vi "rsscope_core_global.vi"() -> ()   [LabVIEW 2018] (continued)
"Descriptive Name"="Amplitude Time Arithmetic Parameter Amptime Type", "Data Type"=0, "Command"="MEAS{Measurement}:AMPT:ARIT:PAR{ArithmeticParameter}:AMPT", "Access"=2, "Range Table"="RsScope_rngAmplitudeTimeArithmeticParameterMeasurementType", "Read Callback"="", "Write Callback"="", "Supported Models"="", "Instrument Options"="", "Flags"=0, "Help"="Selects the amplitude/time arithmetics measurements for the measurment group.\n\nAvailable Repeated Capabilities:\nMeasurement: Meas1, Meas2, Meas3, Meas4, Meas5, Meas6, Meas7, Meas8, Meas9, Meas10\r\nArithmeticParameter: ArithmeticParm1, ArithmeticParm2\r\n\nRemote-control command(s):\nMEASurement<m>:AMPTime:ARIThmetic:PARameter<n>:AMPTime"}, {"Level"=4, "Class Only"=FALSE, "Identifier"="RSSCOPE_ATTR_AMPLITUDE_TIME_ARITHMETIC_PARAMETER_GROUP", "Descriptive Name"="Amplitude Time Arithmetic Parameter Group", "Data Type"=0, "Command"="MEAS{Measurement}:AMPT:ARIT:PAR{ArithmeticParameter}:GRO", "Access"=2, "Range Table"="RsScope_rngSpectrumArithmeticParameterGroup", "Read Callback"="", "Write Callback"="", "Supported Models"="", "Instrument Options"="", "Flags"=0, "Help"="Sets the measurement group for the second operand of the amplitude/time arithmetic measurement.\n\nAvailable Repeated Capabilities:\nMeasurement: Meas1, Meas2, Meas3, Meas4, Meas5, Meas6, Meas7, Meas8, Meas9, Meas10\r\nArithmeticParameter: ArithmeticParm1, ArithmeticParm2\r\n\nRemote-control command(s):\nMEASurement<m>:AMPTime:ARIThmetic:PARameter<n>:GROup"}, {"Level"=4, "Class Only"=FALSE, "Identifier"="RSSCOPE_ATTR_AMPLITUDE_TIME_ARITHMETIC_PARAMETER_MEASUREMENT_SPECTRUM", "Descriptive Name"="Amplitude Time Arithmetic Parameter Measurement Spectrum", "Data Type"=0, "Command"="MEAS{Measurement}:AMPT:ARIT:PAR{ArithmeticParameter}:SPEC", "Access"=2, "Range Table"="RsScope_rngSpectrumArithmeticMeasurementSpectrum", "Read Callback"="", "Write Callback"="", "Supported Models"="", "Instrument Options"="", "Flags"=0, "Help"="Selects the spectrum arithmetics measurements for the measurment group.\n\nAvailable Repeated Capabilities:\nMeasurement: Meas1, Meas2, Meas3, Meas4, Meas5, Meas6, Meas7, Meas8, Meas9, Meas10\r\nArithmeticParameter: ArithmeticParm1, ArithmeticParm2\r\n\nRemote-control command(s):\nMEASurement<m>:AMPTime:ARIThmetic:PARameter<n>:SPECtrum"}, {"Level"=4, "Class Only"=FALSE, "Identifier"="RSSCOPE_ATTR_AMPLITUDE_TIME_ARITHMETIC_OPERATOR", "Descriptive Name"="Amplitude Time Arithmetic Operator", "Data Type"=0, "Command"="MEAS{Measurement}:AMPT:ARIT:OPER", "Access"=2, "Range Table"="RsScope_rngSpectrumArithmeticOperator", "Read Callback"="", "Write Callback"="", "Supported Models"="", "Instrument Options"="", "Flags"=0, "Help"="Selects the operation type to be performed on the selected operands for the amplitude/time arithmetic measurement.\n\nAvailable Repeated Capabilities:\nMeasurement: Meas1, Meas2, Meas3, Meas4, Meas5, Meas6, Meas7, Meas8, Meas9, Meas10\r\n\nRemote-control command(s):\nMEASurement<m>:AMPTime:ARIThmetic:OPERator"}, {"Level"=4, "Class Only"=FALSE, "Identifier"="RSSCOPE_ATTR_AMPLITUDE_TIME_ARITHMETIC_CONSTANT", "Descriptive Name"="Amplitude Time Arithmetic Constant", "Data Type"=1, "Command"="MEAS{Measurement}:AMPT:ARIT:CONS", "Access"=2, "Range Table"="RsScope_rngArithmeticConstant", "Read Callback"="", "Write Callback"="", "Supported Models"="", "Instrument Options"="", "Flags"=0, "Help"="Sets a constant numeric value as the second operand of the amplitude/time arithmetic measurement.\n\nAvailable Repeated Capabilities:\nMeasurement: Meas1, Meas2, Meas3, Meas4, Meas5, Meas6, Meas7, Meas8, Meas9, Meas10\r\n\nRemote-control command(s):\nMEASurement<m>:AMPTime:ARIThmetic:CONStant"}, {"Level"=4, "Class Only"=FALSE, "Identifier"="RSSCOPE_ATTR_AMPLITUDE_TIME_ARITHMETIC_CONSTANT_UNIT", "Descriptive Name"="Amplitude Time Arithmetic Constant Unit", "Data Type"=0, "Command"="MEAS{Measurement}:AMPT:ARIT:COUN", "Access"=2, "Range Table"="RsScope_rngArithmeticOperationType", "Read Callback"="", "Write Callback"="", "Supported Models"="", "Instrument Options"="", "Flags"=0, "Help"="Selects the operation type to be performed on the selected operands for the amplitude/time arithmetic measurement.\n\nAvailable Repeated Capabilities:\nMeasurement: Meas1, Meas2, Meas3, Meas4, Meas5, Meas6, Meas7, Meas8, Meas9, Meas10\r\n\nRemote-control command(s):\nMEASurement<m>:AMPTime:ARIThmetic:COUNit"}, {"Level"=4, "Class Only"=FALSE, "Identifier"="RSSCOPE_ATTR_AMPLITUDE_TIME_ARITHMETIC_CUSTOM_NAME_ENABLED", "Descriptive Name"="Amplitude Time Arithmetic Custom Name Enabled", "Data Type"=3, "Command"="MEAS{Measurement}:AMPT:ARIT:CUNS", "Access"=2, "Range Table"="", "Read Callback"="", "Write Callback"="", "Supported Models"="", "Instrument Options"="", "Flags"=0, "Help"="Enables the use of user-defined custom name for the amplitude/time arithmetic measurement.\n\nAvailable Repeated Capabilities:\nMeasurement: Meas1, Meas2, Meas3, Meas4, Meas5, Meas6, Meas7, Meas8, Meas9, Meas10\r\n\nRemote-control command(s):\nMEASurement<m>:AMPTime:ARIThmetic:CUNState"}, {"Level"=4, "Class Only"=FALSE, "Identifier"="RSSCOPE_ATTR_AMPLITUDE_TIME_ARITHMETIC_CUSTOM_UNIT_ENABLED", "Descriptive Name"="Amplitude Time Arithmetic Custom Unit Enabled", "Data Type"=3, "Command"="MEAS{Measurement}:AMPT:ARIT:CUUS", "Access"=2, "Range Table"="", "Read Callback"="", "Write Callback"="", "Supported Models"="", "Instrument Options"="", "Flags"=0, "Help"="Enables the use of user-defined custom unit for the amplitude/time arithmetic measurement. You can set the unit with RSSCOPE_ATTR_AMPLITUDE_TIME_ARITHMETIC_CUSTOM_UNIT.\n\nAvailable Repeated Capabilities:\nMeasurement: Meas1, Meas2, Meas3, Meas4, Meas5, Meas6, Meas7, Meas8, Meas9, Meas10\r\n\nRemote-control command(s):\nMEASurement<m>:AMPTime:ARIThmetic:CUUState"}, {"Level"=4, "Class Only"=FALSE, "Identifier"="RSSCOPE_ATTR_AMPLITUDE_TIME_ARITHMETIC_CUSTOM_UNIT", "Descriptive Name"="Amplitude Time Arithmetic Custom Unit", "Data Type"=2, "Command"="MEAS{Measurement}:AMPT:ARIT:CUUN", "Access"=2, "Range Table"="", "Read Callback"="", "Write Callback"="", "Supported Models"="", "Instrument Options"="", "Flags"=0, "Help"="Sets a user-defined value of the unit for the amplitude/time arithmetic measurement.\n\nAvailable Repeated Capabilities:\nMeasurement: Meas1, Meas2, Meas3, Meas4, Meas5, Meas6, Meas7, Meas8, Meas9, Meas10\r\n\nRemote-control command(s):\nMEASurement<m>:AMPTime:ARIThmetic:CUUNit"}, {"Level"=3, "Class Only"=TRUE, "Identifier"="", "Descriptive Name"="Source Number", "Data Type"=0, "Command"="", "Access"=0, "Range Table"="", "Read Callback"="", "Write Callback"="", "Supported Models"="", "Instrument Options"="", "Flags"=0, "Help"="Selects Source Number"}, {"Level"=4, "Class Only"=FALSE, "Identifier"="RSSCOPE_ATTR_AMPT_DELAY_LEVEL_SELECTION", "Descriptive Name"="Amplitude Delay Level Selection", "Data Type"=0, "Command"="MEAS{Measurement}:AMPT:DEL{SourceNumber}:LSEL", "Access"=2, "Range Table"="rsscope_rngAmpRefLevSelection", "Read Callback"="", "Write Callback"="", "Supported Models"="", "Instrument Options"="", "Flags"=0, "Help"="Selects the reference level on which the time is measured for each source.\n\nAvailable Repeated Capabilities:\nMeasurement: Meas1, Meas2, Meas3, Meas4, Meas5, Meas6, Meas7, Meas8, Meas9, Meas10\r\nSourceNumber: SN1, SN2, SN3, SN4\r\n\nRemote-control command(s):\nMEASurement<m>:AMPTime:DELay<n>:LSELect"}, {"Level"=4, "Class Only"=FALSE, "Identifier"="RSSCOPE_ATTR_AMPT_DELAY_SLOPE", "Descriptive Name"="Amplitude Delay Slope", "Data Type"=0, "Command"="MEAS{Measurement}:AMPT:DEL{SourceNumber}:SLOP", "Access"=2, "Range Table"="rsscope_rngTriggerSlope", "Read Callback"="", "Write Callback"="", "Supported Models"="", "Instrument Options"="", "Flags"=0, "Help"="Sets the edge of each source, between which the delay is measured.\n\nAvailable Repeated Capabilities:\nMeasurement: Meas1, Meas2, Meas3, Meas4, Meas5, Meas6, Meas7, Meas8, Meas9, Meas10\r\nSourceNumber: SN1, SN2, SN3, SN4\r\n\nRemote-control command(s):\nMEASurement<m>:AMPTime:DELay<n>:SLOPe"}, {"Level"=4, "Class Only"=FALSE, "Identifier"="RSSCOPE_ATTR_AMPT_DELAY_DIRECTION", "Descriptive Name"="Amplitude Delay Direction", "Data Type"=0, "Command"="MEAS{Measurement}:AMPT:DEL{SourceNumber}:DIR", "Access"=2, "Range Table"="rsscope_rngAmplitudeDelayDirection", "Read Callback"="", "Write Callback"="", "Supported Models"="", "Instrument Options"="", "Flags"=0, "Help"="Selects the direction for counting slopes for each source: from the beginning of the waveform, or from the end.\n\nAvailable Repeated Capabilities:\nMeasurement: Meas1, Meas2, Meas3, Meas4, Meas5, Meas6, Meas7, Meas8, Meas9, Meas10\r\nSourceNumber: SN1, SN2, SN3, SN4\r\n\nRemote-control command(s):\nMEASurement<m>:AMPTime:DELay<n>:DIRection"}, {"Level"=4, "Class Only"=FALSE, "Identifier"="RSSCOPE_ATTR_AMPT_DELAY_EDGE_NUMBER", "Descriptive Name"="Amplitude Delay Edge Number", "Data Type"=0, "Command"="MEAS{Measurement}:AMPT:DEL{SourceNumber}:ECO", "Access"=2, "Range Table"="rsscope_rngAmpDelayEdgeNumber", "Read Callback"="", "Write Callback"="", "Supported Models"="", "Instrument Options"="", "Flags"=0, "Help"="Sets the number of the edge that is relevant for delay measurement for each source.\n\nAvailable Repeated Capabilities:\nMeasurement: Meas1, Meas2, Meas3, Meas4, Meas5, Meas6, Meas7, Meas8, Meas9, Meas10\r\nSourceNumber: SN1, SN2, SN3, SN4\r\n\nRemote-control command(s):\nMEASurement<m>:AMPTime:DELay<n>:ECOunt"}, {"Level"=3, "Class Only"=TRUE, "Identifier"="", "Descriptive Name"="Amplitude Measurement Type", "Data Type"=0, "Command"="", "Access"=0, "Range Table"="", "Read Callback"="", "Write Callback"="", "Supported Models"="", "Instrument Options"="", "Flags"=0, "Help"="Selects Amplitude Measurement Type"}, {"Level"=4, "Class Only"=FALSE, "Identifier"="RSSCOPE_ATTR_AMPT_LIMIT_CHECK", "Descriptive Name"="Amplitude Time Limit Check", "Data Type"=0, "Command"="MEAS{Measurement}:AMPT:LCH{AmptMeasurementType}:VAL", "Access"=2, "Range Table"="rsscope_rngLimitCheck", "Read Callback"="", "Write Callback"="", "Supported Models"="", "Instrument Options"="", "Flags"=0, "Help"="Enables or disables limit checking for amplitude vs. time measurements in the specified measurement channel.\n\nAvailable Repeated Capabilities:\nMeasurement: Meas1, Meas2, Meas3, Meas4, Meas5, Meas6, Meas7, Meas8, Meas9, Meas10\r\nAmptMeasurementType: Ampt1, Ampt2, Ampt3, Ampt4, Ampt5, Ampt6, Ampt7, Ampt8, Ampt9, Ampt10, Ampt11, Ampt12, Ampt13, Ampt14, Ampt15, Ampt16, Ampt17, Ampt18, Ampt19, Ampt20, Ampt21, Ampt22, Ampt23, Ampt24, Ampt25, Ampt26, Ampt27, Ampt28, Ampt29, Ampt30, Ampt47, Ampt31, Ampt32, Ampt35, Ampt36, Ampt33, Ampt34, Ampt46, Ampt48, Ampt49\r\n\nRemote-control command(s):\nMEASurement<m>:AMPTime:LCHeck<n>:VALid"}, {"Level"=4, "Class Only"=FALSE, "Identifier"="RSSCOPE_ATTR_AMPLITUDE_TIME_LOWER_LIMIT_VALUE", "Descriptive Name"="Amplitude Time Lower Limit Value", "Data Type"=1, "Command"="MEAS{Measurement}:AMPT:LCH{AmptMeasurementType}:LOW:LIM", "Access"=2, "Range Table"="rsscope_rngAmplitudeLimitValue", "Read Callback"="", "Write Callback"="", "Supported Models"="", "Instrument Options"="", "Flags"=0, "Help"="Define the lower limit for limit checking.\n\nAvailable Repeated Capabilities:\nMeasurement: Meas1, Meas2, Meas3, Meas4, Meas5, Meas6, Meas7, Meas8, Meas9, Meas10\r\nAmptMeasurementType: Ampt1, Ampt2, Ampt3, Ampt4, Ampt5, Ampt6, Ampt7, Ampt8, Ampt9, Ampt10, Ampt11, Ampt12, Ampt13, Ampt14, Ampt15, Ampt16, Ampt17, Ampt18, Ampt19, Ampt20, Ampt21, Ampt22, Ampt23, Ampt24, Ampt25, Ampt26, Ampt27, Ampt28, Ampt29, Ampt30, Ampt47, Ampt31, Ampt32, Ampt35, Ampt36, Ampt33, Ampt34, Ampt46, Ampt48, Ampt49\r\n\nRemote-control command(s):\nMEASurement<m>:AMPTime:LCHeck<n>:LOWer:LIMit"}, {"Level"=4, "Class Only"=FALSE, "Identifier"="RSSCOPE_ATTR_AMPLITUDE_TIME_UPPER_LIMIT_VALUE", "Descriptive Name"="Amplitude Time Upper Limit Value", "Data Type"=1, "Command"="MEAS{Measurement}:AMPT:LCH{AmptMeasurementType}:UPP:LIM", "Access"=2, "Range Table"="rsscope_rngAmplitudeLimitValue", "Read Callback"="", "Write Callback"="", "Supported Models"="", "Instrument Options"="", "Flags"=0, "Help"="Define the upper limit for limit checking.\n\nAvailable Repeated Capabilities:\nMeasurement: Meas1, Meas2, Meas3, Meas4, Meas5, Meas6, Meas7, Meas8, Meas9, Meas10\r\nAmptMeasurementType: Ampt1, Ampt2, Ampt3, Ampt4, Ampt5, Ampt6, Ampt7, Ampt8, Ampt9, Ampt10, Ampt11, Ampt12, Ampt13, Ampt14, Ampt15, Ampt16, Ampt17, Ampt18, Ampt19, Ampt20, Ampt21, Ampt22, Ampt23, Ampt24, Ampt25, Ampt26, Ampt27, Ampt28, Ampt29, Ampt30, Ampt47, Ampt31, Ampt32, Ampt35, Ampt36, Ampt33, Ampt34, Ampt46, Ampt48, Ampt49\r\n\nRemote-control command(s):\nMEASurement<m>:AMPTime:LCHeck<n>:UPPer:LIMit"}, {"Level"=4, "Class Only"=FALSE, "Identifier"="RSSCOPE_ATTR_AMPLITUDE_TIME_LOWER_LIMIT_MARGIN", "Descriptive Name"="Amplitude Time Lower Limit Margin", "Data Type"=1, "Command"="MEAS{Measurement}:AMPT:LCH{AmptMeasurementType}:LOW:MARG", "Access"=2, "Range Table"="rsscope_rngAmplitudeLimitMargin", "Read Callback"="", "Write Callback"="", "Supported Models"="", "Instrument Options"="", "Flags"=0, "Help"="Define the lower margin for the limit check. Margins are not as strict as limits and must be within the valid value range.\n\nAvailable Repeated Capabilities:\nMeasurement: Meas1, Meas2, Meas3, Meas4, Meas5, Meas6, Meas7, Meas8, Meas9, Meas10\r\nAmptMeasurementType: Ampt1, Ampt2, Ampt3, Ampt4, Ampt5, Ampt6, Ampt7, Ampt8, Ampt9, Ampt10, Ampt11, Ampt12, Ampt13, Ampt14, Ampt15, Ampt16, Ampt17, Ampt18, Ampt19, Ampt20, Ampt21, Ampt22, Ampt23, Ampt24, Ampt25, Ampt26, Ampt27, Ampt28, Ampt29, Ampt30, Ampt47, Ampt31, Ampt32, Ampt35, Ampt36, Ampt33, Ampt34, Ampt46, Ampt48, Ampt49\r\n\nRemote-control command(s):\nMEASurement<m>:AMPTime:LCHeck<n>:LOWer:MARGin"}, {"Level"=4, "Class Only"=FALSE, "Identifier"="RSSCOPE_ATTR_AMPLITUDE_TIME_UPPER_LIMIT_MARGIN", "Descriptive Name"="Amplitude Time Upper Limit Margin", "Data Type"=1, "Command"="MEAS{Measurement}:AMPT:LCH{AmptMeasurementType}:UPP:MARG", "Access"=2, "Range Table"="rsscope_rngAmplitudeLimitMargin", "Read Callback"="", "Write Callback"="", "Supported Models"="", "Instrument Options"="", "Flags"=0, "Help"="Define the upper margin for the limit check. Margins are not as strict as limits and must be within the valid value range.\n\nAvailable Repeated Capabilities:\nMeasurement: Meas1, Meas2, Meas3, Meas4, Meas5, Meas6, Meas7, Meas8, Meas9, Meas10\r\nAmptMeasurementType: Ampt1, Ampt2, Ampt3, Ampt4, Ampt5, Ampt6, Ampt7, Ampt8, Ampt9, Ampt10, Ampt11, Ampt12, Ampt13, Ampt14, Ampt15, Ampt16, Ampt17, Ampt18, Ampt19, Ampt20, Ampt21, Ampt22, Ampt23, Ampt24, Ampt25, Ampt26, Ampt27, Ampt28, Ampt29, Ampt30, Ampt47, Ampt31, Ampt32, Ampt35, Ampt36, Ampt33, Ampt34, Ampt46, Ampt48, Ampt49\r\n\nRemote-control command(s):\nMEASurement<m>:AMPTime:LCHeck<n>:UPPer:MARGin"}, {"Level"=2, "Class Only"=TRUE, "Identifier"="", "Descriptive Name"="Jitter Measurement", "Data Type"=0, "Command"="", "Access"=0, "Range Table"="", "Read Callback"="", "Write Callback"="", "Supported Models"="", "Instrument Options"="", "Flags"=0, "Help"="The jitter measurement, option R&S RTO-K12. Jitter describes the timing errors in a system. It is a significant and undesired factor in high-speed serial communication designs because it causes transmission errors."}, {"Level"=3, "Class Only"=FALSE, "Identifier"="RSSCOPE_ATTR_JITTER_MAIN_MEASUREMENT", "Descriptive Name"="Jitter Main Measurement", "Data Type"=0, "Command"="MEAS{Measurement}:MAIN", "Access"=2, "Range Table"="rsscope_rngJitterMainMeasurement", "Read Callback"="", "Write Callback"="", "Supported Models"="", "Instrument Options"="K12", "Flags"=0, "Help"="Defines the jitter main measurement.\n\nAvailable Repeated Capabilities:\nMeasurement: Meas1, Meas2, Meas3, Meas4, Meas5, Meas6, Meas7, Meas8, Meas9, Meas10\r\n\nRemote-control command(s):\nMEASurement<m>:MAIN"}, {"Level"=3, "Class Only"=FALSE, "Identifier"="RSSCOPE_ATTR_JITTER_CLOCK_MEASUREMENT_CYCLE_BEGIN", "Descriptive Name"="Jitter Clock Measurement Cycle Begin", "Data Type"=0, "Command"="MEAS{Measurement}:JITT:CCSL", "Access"=2, "Range Table"="rsscope_rngJitterClockCycleBegin", "Read Callback"="", "Write Callback"="", "Supported Models"="", "Instrument Options"="K12", "Flags"=0, "Help"="Selects the slope at which the periods and thus the jitter is measured.\n\nAvailable Repeated Capabilities:\nMeasurement: Meas1, Meas2, Meas3, Meas4, Meas5, Meas6, Meas7, Meas8, Meas9, Meas10\r\n\nRemote-control command(s):\nMEASurement<m>:JITTer:CCSLope"}, {"Level"=3, "Class Only"=FALSE, "Identifier"="RSSCOPE_ATTR_JITTER_CLOCK_MEASUREMENT_CYCLE_OFFSET", "Descriptive Name"="Jitter Clock Measurement Cycle Offset", "Data Type"=0, "Command"="MEAS{Measurement}:JITT:NCYC", "Access"=2, "Range Table"="rsscope_rngJitterClockCycleOffset", "Read Callback"="", "Write Callback"="", "Supported Models"="", "Instrument Options"="K12", "Flags"=0, "Help"="Sets the distance between the cycles whose periods are taken for the jitter measeurement.\n\nAvailable Repeated Capabilities:\nMeasurement: Meas1, Meas2, Meas3, Meas4, Meas5, Meas6, Meas7, Meas8, Meas9, Meas10\r\n\nRemote-control command(s):\nMEASurement<m>:JITTer:NCYCles"}, {"Level"=3, "Class Only"=FALSE, "Identifier"="RSSCOPE_ATTR_JITTER_CLOCK_MEASUREMENT_PULSE_POLARITY", "Descriptive Name"="Jitter Clock Measurement Pulse Polarity", "Data Type"=0, "Command"="MEAS{Measurement}:JITT:PULS", "Access"=2, "Range Table"="rsscope_rngPolarity", "Read Callback"="", "Write Callback"="", "Supported Models"="", "Instrument Options"="K12", "Flags"=0, "Help"="Sets the polarity of pulses for which the pulse width is measured to obtain the cycle-cycle width and the cycle-cycle duty cycle.\n\nAvailable Repeated Capabilities:\nMeasurement: Meas1, Meas2, Meas3, Meas4, Meas5, Meas6, Meas7, Meas8, Meas9, Meas10\r\n\nRemote-control command(s):\nMEASurement<m>:JITTer:PULSe"}, {"Level"=3, "Class Only"=FALSE, "Identifier"="RSSCOPE_ATTR_JITTER_DATA_MEASUREMENT_CLOCK_MODE", "Descriptive Name"="Jitter Data Measurement Clock Mode", "Data Type"=0, "Command"="MEAS{Measurement}:JITT:CDRM", "Access"=2, "Range Table"="rsscope_rngJitterDataClockMode", "Read Callback"="", "Write Callback"="", "Supported Models"="", "Instrument Options"="K12", "Flags"=0, "Help"="Defines the origin of the clock signal - wether a real clock signal or a clock generated using one of the CDR methods.\n\nAvailable Repeated Capabilities:\nMeasurement: Meas1, Meas2, Meas3, Meas4, Meas5, Meas6, Meas7, Meas8, Meas9, Meas10\r\n\nRemote-control command(s):\nMEASurement<m>:JITTer:CDRMode"}, {"Level"=3, "Class Only"=FALSE, "Identifier"="RSSCOPE_ATTR_JITTER_DATA_MEASUREMENT_DATA_SLOPE", "Descriptive Name"="Jitter Data Measurement Data Slope", "Data Type"=0, "Command"="MEAS{Measurement}:JITT:SOUR1:TIES", "Access"=2, "Range Table"="rsscope_rngTriggerSlope", "Read Callback"="", "Write Callback"="", "Supported Models"="", "Instrument Options"="K12", "Flags"=0, "Help"="Sets the data edges that are used for measurements.\n\nAvailable Repeated Capabilities:\nMeasurement: Meas1, Meas2, Meas3, Meas4, Meas5, Meas6, Meas7, Meas8, Meas9, Meas10\r\n\nRemote-control command(s):\nMEASurement<m>:JITTer:SOURce<n>:TIESlope"}, {"Level"=3, "Class Only"=FALSE, "Identifier"="RSSCOPE_ATTR_JITTER_DATA_MEASUREMENT_CLOCK_SLOPE", "Descriptive Name"="Jitter Data Measurement Clock Slope", "Data Type"=0, "Command"="MEAS{Measurement}:JITT:SOUR2:TIES", "Access"=2, "Range Table"="rsscope_rngTriggerSlope", "Read Callback"="", "Write Callback"="", "Supported Models"="", "Instrument Options"="K12", "Flags"=0, "Help"="Sets the clock and data edges that are used for measurements.\n\nAvailable Repeated Capabilities:\nMeasurement: Meas1, Meas2, Meas3, Meas4, Meas5, Meas6, Meas7, Meas8, Meas9, Meas10\r\n\nRemote-control command(s):\nMEASurement<m>:JITTer:SOURce<n>:TIESlope"}, {"Level"=3, "Class Only"=FALSE, "Identifier"="RSSCOPE_ATTR_JITTER_DATA_MEASUREMENT_UNIT", "Descriptive Name"="Jitter Data Measurement Unit", "Data Type"=0, "Command"="MEAS{Measurement}:JITT:DRUN", "Access"=2, "Range Table"="RsScope_rngJitterDataMeasurementUnit", "Read Callback"="", "Write Callback"="", "Supported Models"="", "Instrument Options"="", "Flags"=0, "Help"="Sets the unit for data rate measurements.\n\nAvailable Repeated Capabilities:\nMeasurement: Meas1, Meas2, Meas3, Meas4, Meas5, Meas6, Meas7, Meas8, Meas9, Meas10\r\n\nRemote-control command(s):\nMEASurement<m>:JITTer:DRUNit"}, {"Level"=3, "Class Only"=FALSE, "Identifier"="RSSCOPE_ATTR_JITTER_DELAY_MEASUREMENT_EDGE_POLARITY", "Descriptive Name"="Jitter Delay Measurement Edge Polarity", "Data Type"=0, "Command"="MEAS{Measurement}:JITT:SKWS", "Access"=2, "Range Table"="rsscope_rngTriggerSlope", "Read Callback"="", "Write Callback"="", "Supported Models"="", "Instrument Options"="K12", "Flags"=0, "Help"="Sets the edge of the first waveform from which the skew delay or phase is measured.\n\nAvailable Repeated Capabilities:\nMeasurement: Meas1, Meas2, Meas3, Meas4, Meas5, Meas6, Meas7, Meas8, Meas9, Meas10\r\n\nRemote-control command(s):\nMEASurement<m>:JITTer:SKWSlope"}, {"Level"=3, "Class Only"=FALSE, "Identifier"="RSSCOPE_ATTR_JITTER_DELAY_MEASUREMENT_RELATIVE_POLARITY", "Descriptive Name"="Jitter Delay Measurement Relative Polarity", "Data Type"=0, "Command"="MEAS{Measurement}:JITT:SKWR", "Access"=2, "Range Table"="rsscope_rngJitterDelayRelativePolarity", "Read Callback"="", "Write Callback"="", "Supported Models"="", "Instrument Options"="K12", "Flags"=0, "Help"="Sets the edge of the second waveform relative to the first waveform.\n\nAvailable Repeated Capabilities:\nMeasurement: Meas1, Meas2, Meas3, Meas4, Meas5, Meas6, Meas7, Meas8, Meas9, Meas10\r\n\nRemote-control command(s):\nMEASurement<m>:JITTer:SKWRelation"}, {"Level"=3, "Class Only"=TRUE, "Identifier"="", "Descriptive Name"="Jitter Measurement Type", "Data Type"=0, "Command"="", "Access"=0, "Range Table"="", "Read Callback"="", "Write Callback"="", "Supported Models"="", "Instrument Options"="", "Flags"=0, "Help"="Selects Jitter Measurement Type"}, {"Level"=4, "Class Only"=FALSE, "Identifier"="RSSCOPE_ATTR_JITTER_LIMIT_CHECK", "Descriptive Name"="Jitter Limit Check", "Data Type"=0, "Command"="MEAS{Measurement}:AMPT:LCH{JitterMeasurementType}:VAL", "Access"=2, "Range Table"="rsscope_rngLimitCheck", "Read Callback"="", "Write Callback"="", "Supported Models"="", "Instrument Options"="K12", "Flags"=0, "Help"="Enables or disables limit checking for amplitude vs. time measurements in the specified measurement channel.\n\nAvailable Repeated Capabilities:\nMeasurement: Meas1, Meas2, Meas3, Meas4, Meas5, Meas6, Meas7, Meas8, Meas9, Meas10\r\nJitterMeasurementType: Jitt1, Jitt2, Jitt3, Jitt4, Jitt5, Jitt6, Jitt7, Jitt8, Jitt9\r\n\nRemote-control command(s):\nMEASurement<m>:AMPTime:LCHeck<n>:VALid"}, {"Level"=4, "Class Only"=FALSE, "Identifier"="RSSCOPE_ATTR_JITTER_LIMIT_LOWER_VALUE", "Descriptive Name"="Jitter Limit Lower Value", "Data Type"=1, "Command"="MEAS{Measurement}:AMPT:LCH{JitterMeasurementType}:LOW:LIM", "Access"=2, "Range Table"="rsscope_rngAmplitudeLimitValue", "Read Callback"="", "Write Callback"="", "Supported Models"="", "Instrument Options"="K12", "Flags"=0, "Help"="Define the lower limit for limit checking, respectively.\n\nAvailable Repeated Capabilities:\nMeasurement: Meas1, Meas2, Meas3, Meas4, Meas5, Meas6, Meas7, Meas8, Meas9, Meas10\r\nJitterMeasurementType: Jitt1, Jitt2, Jitt3, Jitt4, Jitt5, Jitt6, Jitt7, Jitt8, Jitt9\r\n\nRemote-control command(s):\nMEASurement<m>:AMPTime:LCHeck<n>:LOWer:LIMit"}, {"Level"=4, "Class Only"=FALSE, "Identifier"="RSSCOPE_ATTR_JITTER_LIMIT_UPPER_VALUE", "Descriptive Name"="Jitter Limit Upper Value", "Data Type"=1, "Command"="MEAS{Measurement}:AMPT:LCH{JitterMeasurementType}:UPP:LIM", "Access"=2, "Range Table"="rsscope_rngAmplitudeLimitValue", "Read Callback"="", "Write Callback"="", "Supported Models"="", "Instrument Options"="K12", "Flags"=0, "Help"="Define the upper limit for limit checking, respectively.\n\nAvailable Repeated Capabilities:\nMeasurement: Meas1, Meas2, Meas3, Meas4, Meas5, Meas6, Meas7, Meas8, Meas9, Meas10\r\nJitterMeasurementType: Jitt1, Jitt2, Jitt3, Jitt4, Jitt5, Jitt6, Jitt7, Jitt8, Jitt9\r\n\nRemote-control command(s):\nMEASurement<m>:AMPTime:LCHeck<n>:UPPer:LIMit"}, {"Level"=4, "Class Only"=FALSE, "Identifier"="RSSCOPE_ATTR_JITTER_LIMIT_LOWER_MARGIN", "Descriptive Name"="Jitter Limit Lower Margin", "Data Type"=1, "Command"="MEAS{Measurement}:AMPT:LCH{JitterMeasurementType}:LOW:MARG", "Access"=2, "Range Table"="rsscope_rngAmplitudeLimitMargin", "Read Callback"="", "Write Callback"="", "Supported Models"="", "Instrument Options"="K12", "Flags"=0, "Help"="Define the lower and upper margins for the limit check, respectively. Margins are not as strict as limits and must be within the valid value range.\n\nAvailable Repeated Capabilities:\nMeasurement: Meas1, Meas2, Meas3, Meas4, Meas5, Meas6, Meas7, Meas8, Meas9, Meas10\r\nJitterMeasurementType: Jitt1, Jitt2, Jitt3, Jitt4, Jitt5, Jitt6, Jitt7, Jitt8, Jitt9\r\n\nRemote-control command(s):\nMEASurement<m>:AMPTime:LCHeck<n>:LOWer:MARGin"}, {"Level"=4, "Class Only"=FALSE, "Identifier"="RSSCOPE_ATTR_JITTER_LIMIT_UPPER_MARGIN", "Descriptive Name"="Jitter Limit Upper Margin", "Data Type"=1, "Command"="MEAS{Measurement}:AMPT:LCH{JitterMeasurementType}:UPP:MARG", "Access"=2, "Range Table"="rsscope_rngAmplitudeLimitMargin", "Read Callback"="", "Write Callback"="", "Supported Models"="", "Instrument Options"="K12", "Flags"=0, "Help"="Define the upper margins for the limit check, respectively. Margins are not as strict as limits and must be within the valid value range.\n\nAvailable Repeated Capabilities:\nMeasurement: Meas1, Meas2, Meas3, Meas4, Meas5, Meas6, Meas7, Meas8, Meas9, Meas10\r\nJitterMeasurementType: Jitt1, Jitt2, Jitt3, Jitt4, Jitt5, Jitt6, Jitt7, Jitt8, Jitt9\r\n\nRemote-control command(s):\nMEASurement<m>:AMPTime:LCHeck<n>:UPPer:MARGin"}, {"Level"=3, "Class Only"=TRUE, "Identifier"="", "Descriptive Name"="Advanced", "Data Type"=0, "Command"="", "Access"=0, "Range Table"="", "Read Callback"="", "Write Callback"="", "Supported Models"="", "Instrument Options"="", "Flags"=0, "Help"="This class contains methods and attributes for configuring the advanced jitter measurement subsystem (option K133)"}, {"Level"=4, "Class Only"=FALSE, "Identifier"="RSSCOPE_ATTR_ADVANCED_JITTER_ANALYZED_SOURCE", "Descriptive Name"="Advanced Jitter Analyzed Source", "Data Type"=0, "Command"="ADVJ{AdvJitterMeas}:SIGN:SOUR", "Access"=2, "Range Table"="RsScope_rngAdvancedJitterSource", "Read Callback"="", "Write Callback"="", "Supported Models"="", "Instrument Options"="K133|K134", "Flags"=0, "Help"="Selects the source for the advanced jitter analysis.\n\nAvailable Repeated Capabilities:\nAdvJitterMeas: JA1, JA2\r\n\nRemote-control command(s):\nADVJitter<m>:SIGNal:SOURce"}, {"Level"=4, "Class Only"=FALSE, "Identifier"="RSSCOPE_ATTR_ADVANCED_JITTER_SERIAL_STANDARD", "Descriptive Name"="Advanced Jitter Serial Standard", "Data Type"=0, "Command"="ADVJ{AdvJitterMeas}:SIGN:SERS", "Access"=2, "Range Table"="RsScope_rngSoftwareSerialStandard", "Read Callback"="", "Write Callback"="", "Supported Models"="", "Instrument Options"="K133|K134", "Flags"=0, "Help"="Sets the serial standard. Set CUSTOM to adjust the bit rate and the bandwidth manually. The serial standards are available only if the instrument is able to support its maximum nominal bit rate.\n\nAvailable Repeated Capabilities:\nAdvJitterMeas: JA1, JA2\r\n\nRemote-control command(s):\nADVJitter<m>:SIGNal:SERStandard"}, {"Level"=4, "Class Only"=FALSE, "Identifier"="RSSCOPE_ATTR_ADVANCED_JITTER_SIGNAL_TYPE", "Descriptive Name"="Advanced Jitter Signal Type", "Data Type"=0, "Command"="ADVJ{AdvJitterMeas}:SIGN:TYPE", "Access"=2, "Range Table"="RsScope_rngAdvancedJitterSignalType", "Read Callback"="", "Write Callback"="", "Supported Models"="", "Instrument Options"="K133|K134", "Flags"=0, "Help"="Select, if the analyzed signal is a data or clock signal.\n\nAvailable Repeated Capabilities:\nAdvJitterMeas: JA1, JA2\r\n\nRemote-control command(s):\nADVJitter<m>:SIGNal:TYPE"}, {"Level"=4, "Class Only"=FALSE, "Identifier"="RSSCOPE_ATTR_ADVANCED_JITTER_QUICK_START_ANALYSIS", "Descriptive Name"="Advanced Jitter Quick Start Analysis", "Data Type"=4, "Command"="ADVJ{AdvJitterMeas}:SIGN:QUIC", "Access"=1, "Range Table"="", "Read Callback"="", "Write Callback"="", "Supported Models"="", "Instrument Options"="K133|K134", "Flags"=1, "Help"="Starts a quick advanced jitter analysis. Before starting the quick start analysis, set the analyzed source (RSSCOPE_ATTR_ADVANCED_JITTER_ANALYZED_SOURCE) and the signal type (RSSCOPE_ATTR_ADVANCED_JITTER_SIGNAL_TYPE).\n\nThe quick start analysis performs the following:\n- A bit rate estimation is performed on the applied signal.\n- A software CDR of second order is used as reference signal for the jitter analysis.\n- Enables basic measurement Event Count and advanced jitter components: TJ@BER, RJ, TJ, DJ and PJ.\n- In the Result dialog it enables:\n    - Bathtub for total jitter @ BER (TJ@BER).\n    - Step response for the analyzed source signal.\n    - Histogram for RJ, TJ, DJ, DDJ and PJ.\n- Enables the advance jitter measurement analysis.\n\nAvailable Repeated Capabilities:\nAdvJitterMeas: JA1, JA2\r\n\nRemote-control command(s):\nADVJitter<m>:SIGNal:QUICkmeas"}, {"Level"=4, "Class Only"=FALSE, "Identifier"="RSSCOPE_ATTR_ADVANCED_JITTER_REFERENCE_SOURCE", "Descriptive Name"="Advanced Jitter Reference Source", "Data Type"=0, "Command"="ADVJ{AdvJitterMeas}:SIGN:REFS", "Access"=2, "Range Table"="RsScope_rngAdvancedJitterReferenceSource", "Read Callback"="", "Write Callback"="", "Supported Models"="", "Instrument Options"="K133|K134", "Flags"=0, "Help"="Sets that a CDR or clock signal is used as a reference signal.\n\nAvailable Repeated Capabilities:\nAdvJitterMeas: JA1, JA2\r\n\nRemote-control command(s):\nADVJitter<m>:SIGNal:REFSource"}, {"Level"=4, "Class Only"=FALSE, "Identifier"="RSSCOPE_ATTR_ADVANCED_JITTER_REFERENCE_CLOCK_SOURCE", "Descriptive Name"="Advanced Jitter Reference Clock Source", "Data Type"=0, "Command"="ADVJ{AdvJitterMeas}:SIGN:CLKS", "Access"=2, "Range Table"="RsScope_rngAdvancedJitterSource", "Read Callback"="", "Write Callback"="", "Supported Models"="", "Instrument Options"="K133|K134", "Flags"=0, "Help"="Selects the reference source for the clock signal, if RSSCOPE_ATTR_ADVANCED_JITTER_REFERENCE_SOURCE is set to CLOCk.\n\nAvailable Repeated Capabilities:\nAdvJitterMeas: JA1, JA2\r\n\nRemote-control command(s):\nADVJitter<m>:SIGNal:CLKSource"}, {"Level"=4, "Class Only"=FALSE, "Identifier"="RSSCOPE_ATTR_ADVANCED_JITTER_REFERENCE_CDR_SOURCE", "Descriptive Name"="Advanced Jitter Reference CDR Source", "Data Type"=0, "Command"="ADVJ{AdvJitterMeas}:SIGN:CDRM", "Access"=2, "Range Table"="RsScope_rngAdvancedJitterReferenceCDRSource", "Read Callback"="", "Write Callback"="", "Supported Models"="", "Instrument Options"="K133|K134", "Flags"=0, "Help"="Selects the reference source for the CDR signal, if RSSCOPE_ATTR_ADVANCED_JITTER_REFERENCE_SOURCE is set to CDR.\n\nAvailable Repeated Capabilities:\nAdvJitterMeas: JA1, JA2\r\n\nRemote-control command(s):\nADVJitter<m>:SIGNal:CDRMode"}, {"Level"=4, "Class Only"=FALSE, "Identifier"="RSSCOPE_ATTR_ADVANCED_JITTER_REFERENCE_NOMINAL_BITRATE", "Descriptive Name"="Advanced Jitter Reference Nominal Bitrate", "Data Type"=5, "Command"="ADVJ{AdvJitterMeas}:SIGN:BITR", "Access"=2, "Range Table"="RsScope_rngAdvancedJitterNominalBitrate", "Read Callback"="", "Write Callback"="", "Supported Models"="", "Instrument Options"="K133|K134", "Flags"=0, "Help"="Sets the frequency of the feed forward CDR. It corresponds to the data rate of the data stream from which the clock is to be recovered.\n\nAvailable Repeated Capabilities:\nAdvJitterMeas: JA1, JA2\r\n\nRemote-control command(s):\nADVJitter<m>:SIGNal:BITRate"}, {"Level"=4, "Class Only"=FALSE, "Identifier"="RSSCOPE_ATTR_ADVANCED_JITTER_REFERENCE_CLOCK_EDGE", "Descriptive Name"="Advanced Jitter Reference Clock Edge", "Data Type"=0, "Command"="ADVJ{AdvJitterMeas}:SIGN:EDGE", "Access"=2, "Range Table"="RsScope_rngAdvancedJitterClockEdge", "Read Callback"="", "Write Callback"="", "Supported Models"="", "Instrument Options"="K133|K134", "Flags"=0, "Help"="The clock edge sets the point in time when the state of the data signal is checked.\n\nAvailable Repeated Capabilities:\nAdvJitterMeas: JA1, JA2\r\n\nRemote-control command(s):\nADVJitter<m>:SIGNal:EDGE"}, {"Level"=4, "Class Only"=FALSE, "Identifier"="RSSCOPE_ATTR_ADVANCED_JITTER_REFERENCE_CLOCK_SAMPLING_TIME", "Descriptive Name"="Advanced Jitter Reference Clock Sampling Time", "Data Type"=1, "Command"="ADVJ{AdvJitterMeas}:SIGN:SAMT", "Access"=2, "Range Table"="RsScope_rngAdvancedJitterSamplingTime", "Read Callback"="", "Write Callback"="", "Supported Models"="", "Instrument Options"="K133|K134", "Flags"=0, "Help"="Sets a sampling time for the explicit clock signal, an offset for the clock edge in relation to the bit start. The clock edge sets the beginning of the unit interval. The sampling time is a number between 0 and 1. Value 0 sets the clock edge to the beginning of the bit period; value 0.5 sets the clock edge to the middle of the bit period.\n\nAvailable Repeated Capabilities:\nAdvJitterMeas: JA1, JA2\r\n\nRemote-control command(s):\nADVJitter<m>:SIGNal:SAMTime"}, {"Level"=4, "Class Only"=FALSE, "Identifier"="RSSCOPE_ATTR_ADVANCED_JITTER_REFERENCE_CLOCK_MULTIPLIER_FACTOR", "Descriptive Name"="Advanced Jitter Reference Clock Multiplier Factor", "Data Type"=0, "Command"="ADVJ{AdvJitterMeas}:SIGN:CLFF", "Access"=2, "Range Table"="RsScope_rngAdvancedJitterReferenceClockMultiplierFactor", "Read Callback"="", "Write Callback"="", "Supported Models"="", "Instrument Options"="K133|K134", "Flags"=0, "Help"="Sets a clock multiplier factor.\n\nAvailable Repeated Capabilities:\nAdvJitterMeas: JA1, JA2\r\n\nRemote-control command(s):\nADVJitter<m>:SIGNal:CLFFactor"}, {"Level"=4, "Class Only"=FALSE, "Identifier"="RSSCOPE_ATTR_ADVANCED_JITTER_REFERENCE_CLOCK_OFFSET", "Descriptive Name"="Advanced Jitter Reference Clock Offset", "Data Type"=1, "Command"="ADVJ{AdvJitterMeas}:SIGN:CLOF", "Access"=2, "Range Table"="RsScope_rngAdvancedJitterReferenceClockOffset", "Read Callback"="", "Write Callback"="", "Supported Models"="", "Instrument Options"="K133|K134", "Flags"=0, "Help"="Sets a clock offset for the explicit clock signal.\n\nAvailable Repeated Capabilities:\nAdvJitterMeas: JA1, JA2\r\n\nRemote-control command(s):\nADVJitter<m>:SIGNal:CLOFfset"}, {"Level"=4, "Class Only"=FALSE, "Identifier"="RSSCOPE_ATTR_ADVANCED_JITTER_REFERENCE_CLOCK_OFFSET_ESTIMATION", "Descriptive Name"="Advanced Jitter Reference Clock Offset Estimation", "Data Type"=4, "Command"="ADVJ{AdvJitterMeas}:SIGN:CFES", "Access"=1, "Range Table"="", "Read Callback"="", "Write Callback"="", "Supported Models"="", "Instrument Options"="K133|K134", "Flags"=0, "Help"="Executes an estimation of the signal for the clock offset.\n\nAvailable Repeated Capabilities:\nAdvJitterMeas: JA1, JA2\r\n\nRemote-control command(s):\nADVJitter<m>:SIGNal:CFEStimation"}, {"Level"=4, "Class Only"=FALSE, "Identifier"="RSSCOPE_ATTR_ADVANCED_JITTER_REFERENCE_CLOCK_FREQUENCY", "Descriptive Name"="Advanced Jitter Reference Clock Frequency", "Data Type"=1, "Command"="ADVJ{AdvJitterMeas}:SIGN:CLFR", "Access"=2, "Range Table"="RsScope_rngAdvancedJitterReferenceClockFrequency", "Read Callback"="", "Write Callback"="", "Supported Models"="", "Instrument Options"="K133|K134", "Flags"=0, "Help"="Sets the clock frequency for the explicit clock signal.\n\nAvailable Repeated Capabilities:\nAdvJitterMeas: JA1, JA2\r\n\nRemote-control command(s):\nADVJitter<m>:SIGNal:CLFRequency"}, {"Level"=4, "Class Only"=FALSE, "Identifier"="RSSCOPE_ATTR_ADVANCED_JITTER_REFERENCE_CLOCK_FREQ_ESTIMATION", "Descriptive Name"="Advanced Jitter Reference Clock Freq Estimation", "Data Type"=4, "Command"="ADVJ{AdvJitterMeas}:SIGN:CLES", "Access"=1, "Range Table"="", "Read Callback"="", "Write Callback"="", "Supported Models"="", "Instrument Options"="K133|K134", "Flags"=0, "Help"="Executes an estimation of the signal for the clock frequency.\n\nAvailable Repeated Capabilities:\nAdvJitterMeas: JA1, JA2\r\n\nRemote-control command(s):\nADVJitter<m>:SIGNal:CLEStimation"}, {"Level"=4, "Class Only"=FALSE, "Identifier"="RSSCOPE_ATTR_ADVANCED_JITTER_REFERENCE_CLOCK_DATA_RATE", "Descriptive Name"="Advanced Jitter Reference Clock Data Rate", "Data Type"=1, "Command"="ADVJ{AdvJitterMeas}:SIGN:DATR?", "Access"=0, "Range Table"="RsScope_rngAdvancedJitterReferenceClockDataRate", "Read Callback"="", "Write Callback"="", "Supported Models"="", "Instrument Options"="K133|K134", "Flags"=0, "Help"="Displays the calculated data rate of the explicit clock signal.\n\nAvailable Repeated Capabilities:\nAdvJitterMeas: JA1, JA2\r\n\nRemote-control command(s):\nADVJitter<m>:SIGNal:DATRate?"}, {"Level"=4, "Class Only"=FALSE, "Identifier"="RSSCOPE_ATTR_ADVANCED_JITTER_REFERENCE_UI_OFFSET", "Descriptive Name"="Advanced Jitter Reference UI Offset", "Data Type"=1, "Command"="ADVJ{AdvJitterMeas}:SIGN:SAMT", "Access"=2, "Range Table"="RsScope_rngUIOffset", "Read Callback"="", "Write Callback"="", "Supported Models"="", "Instrument Options"="K133|K134", "Flags"=0, "Help"="Defines the position of the last bit of the bit pattern to be triggered on, relative to the trigger time. The unit interval offset is a number between 0 and 1:\n- Value 0: start/left edge of the last bit\n- Value 0.5: middle of the last bit\n- Value 1: end/right edge of the last bit\n\nAvailable Repeated Capabilities:\nAdvJitterMeas: JA1, JA2\r\n\nRemote-control command(s):\nADVJitter<m>:SIGNal:SAMTime"}, {"Level"=4, "Class Only"=TRUE, "Identifier"="", "Descriptive Name"="Gating", "Data Type"=0, "Command"="", "Access"=0, "Range Table"="", "Read Callback"="", "Write Callback"="", "Supported Models"="", "Instrument Options"="", "Flags"=0, "Help"="This class contains attribute and methods for configuring gating setup in the advanced jitter measurement subsystem (option K133)"}, {"Level"=5, "Class Only"=FALSE, "Identifier"="RSSCOPE_ATTR_ADVANCED_JITTER_GATING_ENABLED", "Descriptive Name"="Advanced Jitter Gating Enabled", "Data Type"=3, "Command"="ADVJ{AdvJitterMeas}:SIGN:GATE:STAT", "Access"=2, "Range Table"="", "Read Callback"="", "Write Callback"="", "Supported Models"="", "Instrument Options"="K133|K134", "Flags"=0, "Help"="Enables the gating setup for the advanced jitter analysis.\n\nAvailable Repeated Capabilities:\nAdvJitterMeas: JA1, JA2\r\n\nRemote-control command(s):\nADVJitter<m>:SIGNal:GATE:STATe"}, {"Level"=5, "Class Only"=FALSE, "Identifier"="RSSCOPE_ATTR_ADVANCED_JITTER_GATING_COUPLING_MODE", "Descriptive Name"="Advanced Jitter Gating Coupling Mode", "Data Type"=0, "Command"="ADVJ{AdvJitterMeas}:SIGN:GATE:COUP", "Access"=2, "Range Table"="RsScope_rngAdvancedJitterGateCouplingMode", "Read Callback"="", "Write Callback"="", "Supported Models"="", "Instrument Options"="K133|K134", "Flags"=0, "Help"="Sets if the gate is coupled to the zoom or cursor.\n\nAvailable Repeated Capabilities:\nAdvJitterMeas: JA1, JA2\r\n\nRemote-control command(s):\nADVJitter<m>:SIGNal:GATE:COUPling"}, {"Level"=5, "Class Only"=FALSE, "Identifier"="RSSCOPE_ATTR_ADVANCED_JITTER_GATING_COUPLED_CURSOR", "Descriptive Name"="Advanced Jitter Gating Coupled Cursor", "Data Type"=0, "Command"="ADVJ{AdvJitterMeas}:SIGN:GATE:CURS", "Access"=2, "Range Table"="rsscope_rngCursor", "Read Callback"="", "Write Callback"="", "Supported Models"="", "Instrument Options"="K133|K134", "Flags"=0, "Help"="Sets the cursor the gate is coupled to, if RSSCOPE_ATTR_ADVANCED_JITTER_GATING_COUPLING_MODE is set to CURSor.\n\nAvailable Repeated Capabilities:\nAdvJitterMeas: JA1, JA2\r\n\nRemote-control command(s):\nADVJitter<m>:SIGNal:GATE:CURSor"}, {"Level"=5, "Class Only"=FALSE, "Identifier"="RSSCOPE_ATTR_ADVANCED_JITTER_GATING_COUPLED_ZOOM_DIAGRAM", 
